vi "Read_indicator_in_stream.vi"(10 "Required_indicatorl_name":string="Slide", 11 "reference":refnum<vi>) -> (2 "Value":variant, 3 "reference out":refnum<vi>)   [LabVIEW 2012]
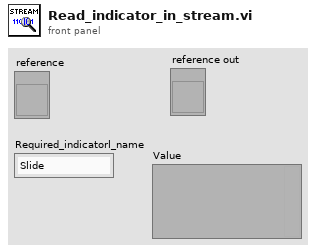
[diagram p1: front panel]
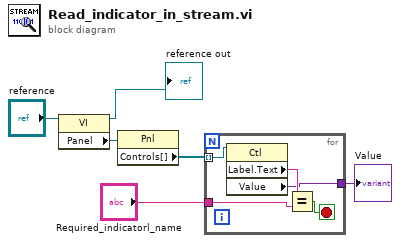
[diagram p0: block diagram]
diagram:
  n1 = property class="VI"(reference="reference") -> (reference out=→"reference out":refnum<vi>, "Panel"=w4:refnum<vi>)  [unwired: 1 in, 1 out]
  n2 = property class="Pnl"(reference=w4) -> ("Controls[]"=w5:refnum<vi>[])  [unwired: 1 in, 2 out]
  n3 = for {
    tunnel: w5 -> [w10] mode=indexing
    tunnel: [w9] -> w1
    tunnel: "Required_indicatorl_name" -> [w7]
    stop <- w8 stop-if-true
    n4 = property class="Ctl"(reference=w10) -> ("Label.Text"=w11:string, "Value"=w9:variant)  [unwired: 1 in, 2 out]
    n5 = Equal?(x=w11, y=w7) -> (x = y?=w8:bool)
  }
  "Value" <- w1
